vi "Tester.vi"() -> ()   [LabVIEW 2019]
uses:
  ControlPlans/ControlPlan.ctl
  ByteGSAPIBase.lvclass
panel:
  out "Array":T1[](array[typedef])
  out "error out":errorcluster
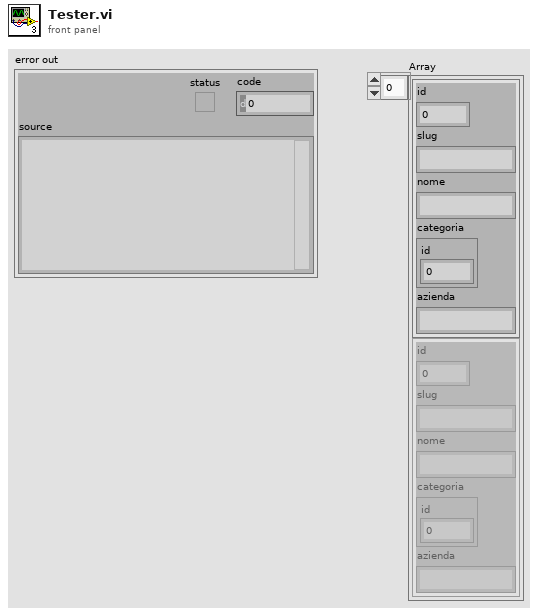
[diagram p1: front panel]
types:
  T1 = typedef "ByteGSWebAPI.lvlib/ByteGSAPIBase.lvclass/ControlPlan.ctl" = cluster{"id":i32, "slug":string, "nome":string, "categoria":cluster{"id":i32}, "azienda":string}
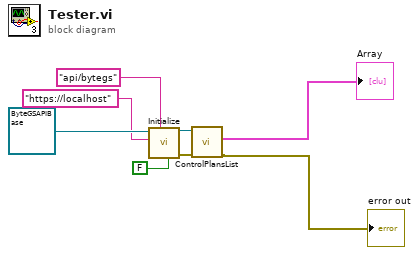
[diagram p0: block diagram]
diagram:
  n1 = call-dynamic "Initialize.vi"("verify server (true)"=FALSE, "API Root"="api/bytegs", "Base URL"="https://localhost", "ByteGSAPIBase in"=refnum<class "ByteGSAPIBase.lvclass"> refnum ("ByteGSWebAPI.lvlib:ByteGSAPIBase.lvclass")) -> ("error out"=w3:errorcluster, "ByteGSAPIBase out"=w4:refnum<class "ByteGSAPIBase.lvclass">)  [unwired: 6 in]
  n2 = call-dynamic "ControlPlansList.vi"("error in (no error)"=w3, "ByteGSAPIBase in"=w4) -> ("error out"=→"error out":errorcluster, "Control plans"=→"Array":T1[])  [unwired: 7 in, 1 out]
